vi "Read.vi"(8 "error in (no error)":errorcluster, 9 "Timeout (1s)":dbl[unit]=1.0, 11 "PVConnection in":refnum<class "SVConnection.lvclass">) -> (0 "error out":errorcluster, 1 "timed out":bool, 2 "PV":refnum<class "PV.lvclass">, 3 "PVConnection out":refnum<class "SVConnection.lvclass">)   [LabVIEW 2013, in "CS++ProcessVariables.lvlib" / "SVConnection.lvclass"]
doc: "Read a process varibale."
uses:
  SVConnection.lvclass
  ProcessVariable/PV.lvclass
  SVConnection.lvclass/SVConnection.ctl
  PVConnection/PVConnection.lvclass/PVConnection.ctl
  ProcessVariable/PV.lvclass/PV.ctl
  ProcessVariable/Write Data.vi
  ProcessVariable/Write Error.vi
  ProcessVariable/Write Timestamp.vi
  ProcessVariable/Write status.vi
  ProcessVariable/Write Quality.vi
  PVConnection/PVConnection.lvclass
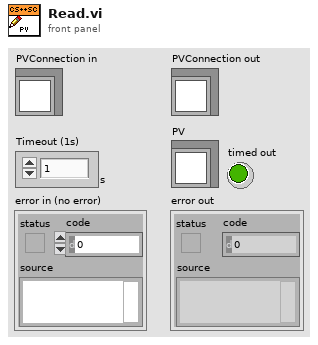
[diagram p1: front panel]
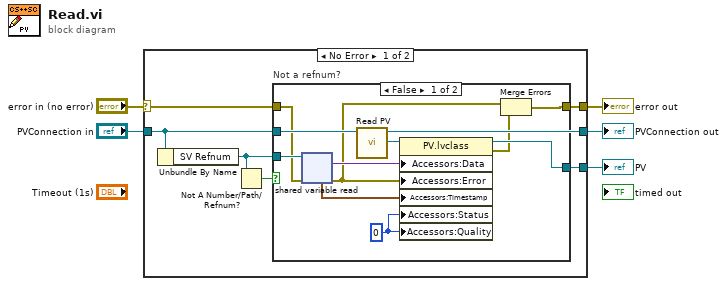
[diagram p0: block diagram]
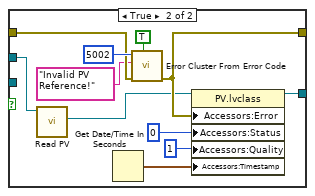
[diagram p2: hidden frame]
diagram:
  n1 = case shown="No Error" "error in (no error)" {
    selector: "error in (no error)" -> [w8 w34]
    tunnel: [w11 w34] -> w2
    tunnel: [w7 w35] -> w3
    tunnel: "PVConnection in" -> [w7 w35]
    tunnel: [w6 _] -> w1
    frame No Error {
      n2 = Unbundle By Name(w7) -> ("SV Refnum"=w9:refnum<k21>)
      n3 = Not A Number/Path/Refnum?(number/path/refnum=w9) -> (NaN/Path/Refnum?=w10:bool)
      n4 = case "Not a refnum?" shown="False" w10 {
        tunnel: w9 -> [w22 _]
        tunnel: w8 -> [w21 w31]
        tunnel: [w14 w27] -> w11
        tunnel: w7 -> [w20 w29]
        tunnel: [w16 w28] -> w6
        frame False {
          w17 = u32 0 ("status")
          n5 = shared-variable-read(w22, w21) -> (w13:errorcluster, w19:variant, w18:timestamp)  [unwired: 1 out]
          n6 = call "Read PV.vi"("PVConnection in"=w20) -> ("PV"=w12:refnum<class "PV.lvclass">)  [unwired: 8 in, 2 out]
          n7 = property class="PV.lvclass"(reference=w12, "Accessors:Data"=w19, "Accessors:Error"=w13, "Accessors:Timestamp"=w18, "Accessors:Status"=w17, "Accessors:Quality"=w17) -> (reference out=w16:refnum<class "PV.lvclass">, error out=w15:errorcluster)  [unwired: 1 in]
          n8 = Merge Errors(w13, w15) -> (w14:errorcluster)
        }
        frame True {
          n9 = call "Read PV.vi"("PVConnection in"=w29) -> ("PV"=w23:refnum<class "PV.lvclass">)  [unwired: 8 in, 2 out]
          n10 = Get Date/Time In Seconds() -> (seconds since 1Jan1904=w24:timestamp)
          n11 = call <vilib>:"Error Cluster From Error Code.vi"("show call chain? (False)"=TRUE, "error in (no error)"=w31, "error message (\"\")"="Invalid PV Reference!" ("error message (\"\")"), "error code (0)"=5002) -> ("error out"=w27:errorcluster)  [unwired: 5 in]
          n12 = property class="PV.lvclass"(reference=w23, "Accessors:Error"=w27, "Accessors:Status"=u32 0 ("status"), "Accessors:Quality"=u64 1 ("quality"), "Accessors:Timestamp"=w24) -> (reference out=w28:refnum<class "PV.lvclass">)  [unwired: 1 in, 1 out]
        }
      }
    }
    frame Error {
    }
  }
  "error out" <- w2
  "PVConnection out" <- w3
  "PV" <- w1
